vi "Rectify Image.vi"   [LabVIEW 2020, in "image.lvlib" / "ImageRectifier.lvclass"]
uses:
  ImageRectifier.lvclass
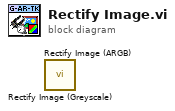
[diagram p0: block diagram]
diagram:
  n1 = call "Rectify Image (Greyscale).vi"() -> ()  [unwired: 9 in, 3 out]
  n2 = call "Rectify Image (ARGB).vi"() -> ()  [unwired: 9 in, 3 out]
